vi "Begin - Davis.vi"(8 "error in":errorcluster) -> (0 "error out":errorcluster)   [LabVIEW 2018]
doc: "Called before other user functions, this VI is expected to open initial I/O refnums, load in file data, and do all program initialization. Notice that the <B>error out</B> terminal is simply used for data flow. Wiring it to other structures or subVIs ensures that this VI runs first."
uses:
  <vilib>/Rock Robotics/WPI/ThirdParty/Phoenix-LabVIEW/Motor Controller/Controls/CTRE_Phoenix_MotorControl_EnhancedMotorControllerConfigurables.ctl
  <vilib>/Rock Robotics/WPI/ThirdParty/Phoenix-LabVIEW/Motor Controller/Controls/CTRE_Phoenix_MotorControl_BaseConfigurables.ctl
  <vilib>/Rock Robotics/WPI/ThirdParty/Phoenix-LabVIEW/Motor Controller/Controls/CTRE_Phoenix_MotorControl_VelocityMeasurementPeriod.ctl
  <vilib>/Rock Robotics/WPI/ThirdParty/Phoenix-LabVIEW/Motor Controller/Controls/CTRE_Phoenix_MotorControl_SlotStructure.ctl
  <vilib>/Rock Robotics/WPI/ThirdParty/Phoenix-LabVIEW/Motor Controller/Controls/CTRE_Phoenix_MotorControl_FilterStruct.ctl
  <vilib>/Rock Robotics/WPI/ThirdParty/Phoenix-LabVIEW/Motor Controller/Controls/CTRE_Phoenix_MotorControl_RemoteSourceType.ctl
  <vilib>/Rock Robotics/WPI/ThirdParty/Phoenix-LabVIEW/Controls/CTRE_Phoenix_CustomParamConfiguration.ctl
  <vilib>/Rock Robotics/WPI/ThirdParty/Phoenix-LabVIEW/Motor Controller/Controls/CTRE_Phoenix_MotorControl_FeedbackDevice.ctl
  <vilib>/Rock Robotics/WPI/ThirdParty/Phoenix-LabVIEW/Motor Controller/Controls/CTRE_Phoenix_MotorControl_SensorTermFeedbackDevice_Enhanced.ctl
  <vilib>/Rock Robotics/WPI/ThirdParty/Phoenix-LabVIEW/Motor Controller/Controls/CTRE_Phoenix_MotorControl_LimitSwitchNormal.ctl
  <vilib>/Rock Robotics/WPI/ThirdParty/Phoenix-LabVIEW/Motor Controller/Controls/CTRE_Phoenix_MotorControl_LimitSwitchSource_Local.ctl
  <vilib>/Rock Robotics/WPI/DriverStation/WPI_DriverStationRobotMode2.ctl
  <vilib>/Rock Robotics/WPI/ThirdParty/Phoenix-LabVIEW/Motor Controller/Controls/CTRE_Phoenix_MotorControl_ControlMode.ctl
  <vilib>/Rock Robotics/WPI/Solenoid/WPI_SolenoidChannel.ctl
  <vilib>/Rock Robotics/WPI/SafetyOutput/WPI_SafetyOutputConfigMenu.ctl
  <vilib>/Rock Robotics/WPI/Joystick/WPI_JoystickDeviceEnum.ctl
  <vilib>/Rock Robotics/SystemInterfaces/DIO/FPGA_DIOPWMChannel.ctl
  <vilib>/Rock Robotics/SystemInterfaces/DIO/FPGA_DIOChannel.ctl
  Robot Global Data.vi
  <vilib>/Rock Robotics/Network Tables/NT Write String Array.vi
  <vilib>/Rock Robotics/WPI/Solenoid/WPI_SolenoidOpenDouble.vi
  <vilib>/Rock Robotics/WPI/Switch/WPI_SwitchOpenLimit.vi
  <vilib>/Rock Robotics/WPI/MotorControl/WPI_MotorControlOpen Victor.vi
  <vilib>/Rock Robotics/WPI/RobotDrive/WPI_RobotDriveOpen2MotorWithExistingMotors.vi
  <vilib>/Rock Robotics/WPI/MotorControl/WPI_MotorControlOpen SPARK.vi
  <vilib>/Rock Robotics/WPI/RobotDrive/WPI_RobotDriveOpen2MotorWithTalon.vi
panel:
  in  "Enhanced Motor Controller Configurables":T1={"Base Configurables"={"openLoopRamp"=0.0, "closedLoopRamp"=0.0, "peakOutputForward"=1.0, "peakOutputReverse"=-1.0, "nominalOutputForward"=0.0, "nominalOutputReverse"=0.0, "neutralDeadband"=0.04, "voltageCompSaturation"=0.0, "voltageMeasurementFilter"=32, "velocityMeasurementPeriod"=100, "velocityMeasurementWindow"=64, "forwardSoftLimitThreshold"=0, "reverseSoftLimitThreshold"=0, "forwardSoftLimitEnable"=FALSE, "reverseSoftLimitEnable"=FALSE, "slot0"={"P"=0.0, "I"=0.0, "D"=0.0, "F"=0.0, "integralZone"=0.0, "allowableClosedLoopError"=0, "maxIntegralAccumulator"=0.0, "closedLoopPeakOutput"=1.0, "closedLoopPeriod"=1}, "slot1"={"P"=0.0, "I"=0.0, "D"=0.0, "F"=0.0, "integralZone"=0.0, "allowableClosedLoopError"=0, "maxIntegralAccumulator"=0.0, "closedLoopPeakOutput"=1.0, "closedLoopPeriod"=1}, "slot2"={"P"=0.0, "I"=0.0, "D"=0.0, "F"=0.0, "integralZone"=0.0, "allowableClosedLoopError"=0, "maxIntegralAccumulator"=0.0, "closedLoopPeakOutput"=1.0, "closedLoopPeriod"=1}, "slot3"={"P"=0.0, "I"=0.0, "D"=0.0, "F"=0.0, "integralZone"=0.0, "allowableClosedLoopError"=0, "maxIntegralAccumulator"=0.0, "closedLoopPeakOutput"=1.0, "closedLoopPeriod"=1}, "auxPIDPolarity"=FALSE, "remoteFilter0"={"remoteSensorDeviceID"=0, "remoteSensorSource"=enum."Off"}, "remoteFilter1"={"remoteSensorDeviceID"=0, "remoteSensorSource"=enum."Off"}, "motionCruiseVelocity"=0, "motionAcceleration"=0, "motionProfileTrajectoryPeriod"=0, "feedbackNotContinuous"=FALSE, "remoteSensorClosedLoopDisableNeutralOnLOS"=FALSE, "clearPositionOnLimitF"=FALSE, "clearPositionOnLimitR"=FALSE, "clearPositionOnQuadIdx"=FALSE, "limitSwitchDisableNeutralOnLOS"=FALSE, "softLimitDisableNeutralOnLOS"=FALSE, "pulseWidthPeriod_EdgesPerRot"=1, "pulseWidthPeriod_FilterWindowSz"=1, "customParam"={"customParam0"=0, "customParam1"=0}, "trajectoryInterpolationEnable"=TRUE}, "primaryPID"={"selectedFeedbackCoefficient"=1.0, "selectedFeedbackSensor"=0}, "auxiliaryPID"={"selectedFeedbackCoefficient"=1.0, "selectedFeedbackSensor"=0}, "sum0Term"=0, "sum1Term"=0, "diff0Term"=0, "diff1Term"=0, "forwardLimitSwitchNormal"=enum."Normally Open", "reverseLimitSwitchNormal"=enum."Normally Open", "forwardLimitSwitchDeviceID"=0, "reverseLimitSwitchDeviceID"=0, "forwardLimitSwitchSource"=enum."Feedback Connector", "reverseLimitSwitchSource"=enum."Feedback Connector", "peakCurrentLimit"=1, "peakCurrentDuration"=1, "continuousCurrentLimit"=1} {"diff1Term" items=["QuadEncoder"=0, "Analog"=2, "Tachometer"=4, "Pulse Width Encoded Position"=8, "Remote Source 0"=11, "Remote Source 1"=12, "Software Emulated"=15]; "diff0Term" items=["QuadEncoder"=0, "Analog"=2, "Tachometer"=4, "Pulse Width Encoded Position"=8, "Remote Source 0"=11, "Remote Source 1"=12, "Software Emulated"=15]; "sum1Term" items=["QuadEncoder"=0, "Analog"=2, "Tachometer"=4, "Pulse Width Encoded Position"=8, "Remote Source 0"=11, "Remote Source 1"=12, "Software Emulated"=15]; "sum0Term" items=["QuadEncoder"=0, "Analog"=2, "Tachometer"=4, "Pulse Width Encoded Position"=8, "Remote Source 0"=11, "Remote Source 1"=12, "Software Emulated"=15]; "auxiliaryPID"."selectedFeedbackSensor" items=["QuadEncoder"=0, "Analog"=2, "Tachometer"=4, "Pulse Width Encoded Position"=8, "Sensor Sum (S0 + S1)"=9, "Sensor Difference (D0 - D1)"=10, "Remote Source 0"=11, "Remote Source 1"=12, "Software Emulated"=15]; "primaryPID"."selectedFeedbackSensor" items=["QuadEncoder"=0, "Analog"=2, "Tachometer"=4, "Pulse Width Encoded Position"=8, "Sensor Sum (S0 + S1)"=9, "Sensor Difference (D0 - D1)"=10, "Remote Source 0"=11, "Remote Source 1"=12, "Software Emulated"=15]; "Base Configurables"."velocityMeasurementPeriod" items=["Period_1ms"=1, "Period_2ms"=2, "Period_5ms"=5, "Period_10ms"=10, "Period_20ms"=20, "Period_25ms"=25, "Period_50ms"=50, "Period_100ms"=100]}
  # "Sum and Diff terms are ways to select more than one sensor as a feedback device. \n Sum 0 is the first feedback device to be used for the Sum term.\n Sum 1 is the feedback device to be added to Sum 0 for the Sum term.\n Diff 0 and Diff 1 work in a similar manner."
  # "These are only applicable\nif using a remote limit switch.\n\nLocal limit switches/no limit\nswitches do not use this."
  # "Current is below Continuous threshold AND\n\n(Requested output is weaker** than applied motor\noutput OR is in the opposite direction).\n/\nMotor output is set to requested output."
  # "Current is above Peak* Threshold for Peak Duration.\n/\nReduce motor output (towards neutral)."
  # "Current is below Continuous threshold.\n/\nRamp motor output towards requested output."
  # "Current is above Continuous threshold.\n/\nReduce motor output (towards neutral)."
  # "Current Limiting is NOT enabled\nby default.\nCall this VI to enable."
  # "*If the configured Peak Threshold is less than the Continuous Threshold, the applied Peak Threshold is set equal to the Configured Continuous Threshold in firmware.\n** Both requested output and applied motor output are in the same direction, and requested output is closer to neutral."
  # "False: Primary Output = PID[0] + PID[1]  ---  Auxiliary Output = PID[0] - PID[1]\nTrue:  Primary Output = PID[0] - PID[1] --- Auxiliary Output = PID[0] + PID[1]"
  # "Enable the motion profile executor to perform linear interpolation between profile points.  Defaults to True."
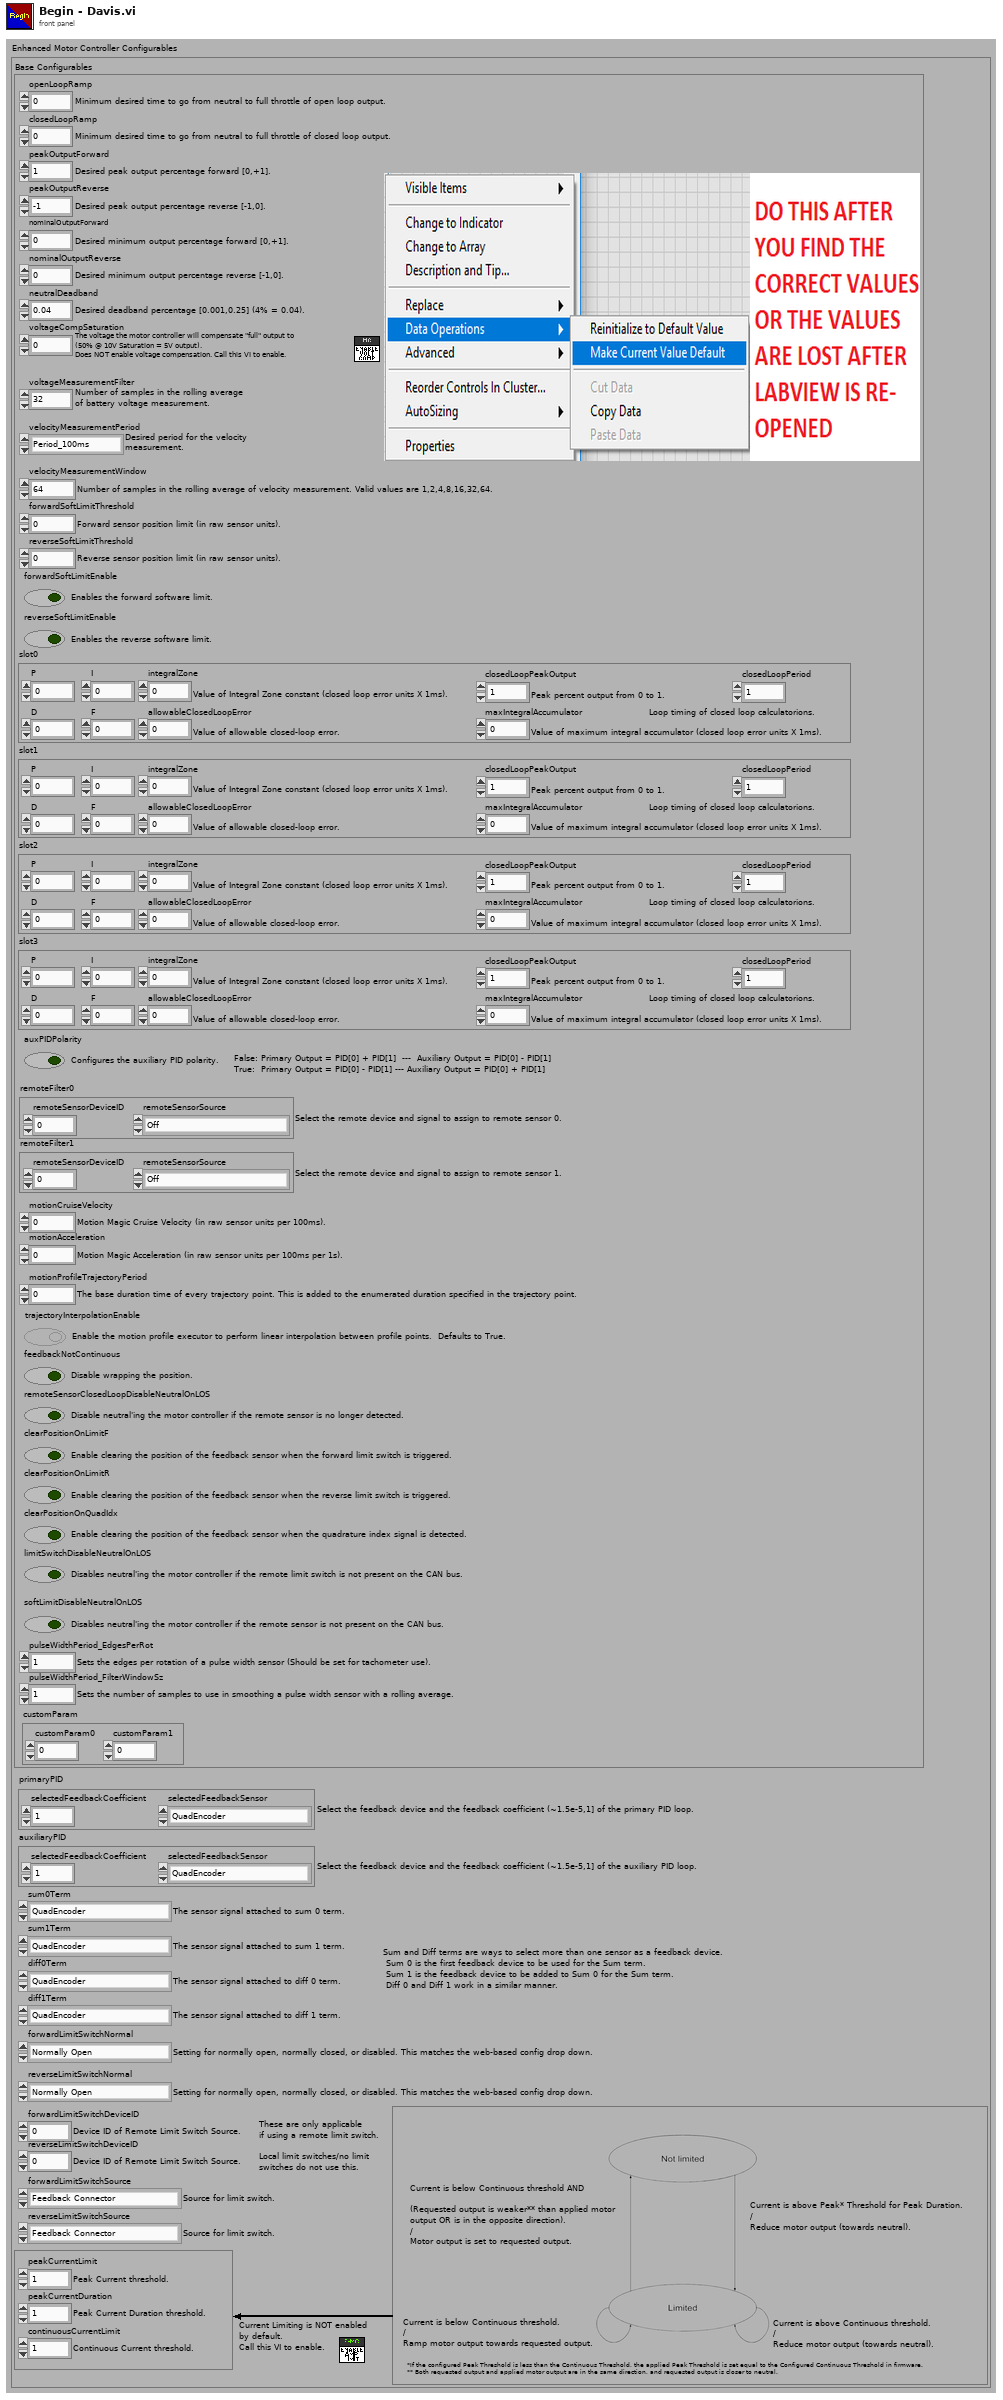
[diagram p1: front panel]
types:
  T1 = typedef "CTRE_Phoenix_MotorControl_EnhancedMotorControllerConfigurables.ctl" = cluster{"Base Configurables":T2, "primaryPID":cluster{"selectedFeedbackCoefficient":dbl, "selectedFeedbackSensor":T8}, "auxiliaryPID":cluster{"selectedFeedbackCoefficient":dbl, "selectedFeedbackSensor":T8}, "sum0Term":T9, "sum1Term":T9, "diff0Term":T9, "diff1Term":T9, "forwardLimitSwitchNormal":T10, "reverseLimitSwitchNormal":T10, "forwardLimitSwitchDeviceID":i32, "reverseLimitSwitchDeviceID":i32, "forwardLimitSwitchSource":T11, "reverseLimitSwitchSource":T11, "peakCurrentLimit":i32, "peakCurrentDuration":i32, "continuousCurrentLimit":i32}
  T2 = typedef "CTRE_Phoenix_MotorControl_BaseConfigurables.ctl" = cluster{"openLoopRamp":dbl, "closedLoopRamp":dbl, "peakOutputForward":dbl, "peakOutputReverse":dbl, "nominalOutputForward":dbl, "nominalOutputReverse":dbl, "neutralDeadband":dbl, "voltageCompSaturation":dbl, "voltageMeasurementFilter":i32, "velocityMeasurementPeriod":T3, "velocityMeasurementWindow":i32, "forwardSoftLimitThreshold":i32, "reverseSoftLimitThreshold":i32, "forwardSoftLimitEnable":bool, "reverseSoftLimitEnable":bool, "slot0":T4, "slot1":T4, "slot2":T4, "slot3":T4, "auxPIDPolarity":bool, "remoteFilter0":T5, "remoteFilter1":T5, "motionCruiseVelocity":i32, "motionAcceleration":i32, "motionProfileTrajectoryPeriod":i32, "feedbackNotContinuous":bool, "remoteSensorClosedLoopDisableNeutralOnLOS":bool, "clearPositionOnLimitF":bool, "clearPositionOnLimitR":bool, "clearPositionOnQuadIdx":bool, "limitSwitchDisableNeutralOnLOS":bool, "softLimitDisableNeutralOnLOS":bool, "pulseWidthPeriod_EdgesPerRot":i32, "pulseWidthPeriod_FilterWindowSz":i32, "customParam":T7, "trajectoryInterpolationEnable":bool}
  T3 = typedef "CTRE_Phoenix_MotorControl_VelocityMeasurementPeriod.ctl" = u16
  T4 = typedef "CTRE_Phoenix_MotorControl_SlotStructure.ctl" = cluster{"P":dbl, "I":dbl, "D":dbl, "F":dbl, "integralZone":dbl, "allowableClosedLoopError":i32, "maxIntegralAccumulator":dbl, "closedLoopPeakOutput":dbl, "closedLoopPeriod":i32}
  T5 = typedef "CTRE_Phoenix_MotorControl_FilterStruct.ctl" = cluster{"remoteSensorDeviceID":u8, "remoteSensorSource":T6}
  T6 = typedef "CTRE_Phoenix_MotorControl_RemoteSourceType.ctl" = enum16{"Off", "Talon SRX Selected Sensor", "Pigeon IMU Yaw", "Pigeon IMU Pitch", "Pigeon IMU Roll", "CANifier Quadrature", "CANifier PWM Input 0", "CANifier PWM Input 1", "CANifier PWM Input 2", "CANifier PWM Input 3", "Gadgeteer Pigeon Yaw", "Gadgeteer Pigeon Pitch", "Gadgeteer Pigeon Roll"}
  T7 = typedef "CTRE_Phoenix_CustomParamConfiguration.ctl" = cluster{"customParam0":i32, "customParam1":i32}
  T8 = typedef "CTRE_Phoenix_MotorControl_FeedbackDevice.ctl" = i8
  T9 = typedef "CTRE_Phoenix_MotorControl_SensorTermFeedbackDevice_Enhanced.ctl" = i8
  T10 = typedef "CTRE_Phoenix_MotorControl_LimitSwitchNormal.ctl" = enum16{"Normally Open", "Normally Closed", "Disabled"}
  T11 = typedef "CTRE_Phoenix_MotorControl_LimitSwitchSource_Local.ctl" = enum16{"Feedback Connector", "Remote Talon SRX", "Remote CANifier", "Deactivated"}
  T12 = typedef "WPI_SafetyOutputConfigMenu.ctl" = enum16{"Enable", "Disable"}
  T13 = typedef "WPI_SolenoidChannel.ctl" = enum8{"Solenoid 0", "Solenoid 1", "Solenoid 2", "Solenoid 3", "Solenoid 4", "Solenoid 5", "Solenoid 6", "Solenoid 7", "Invalid"}
  T14 = typedef "FPGA_DIOPWMChannel.ctl" = enum8{"PWM 0", "PWM 1", "PWM 2", "PWM 3", "PWM 4", "PWM 5", "PWM 6", "PWM 7", "PWM 8", "PWM 9", "PWM MXP 0", "PWM MXP 1", "PWM MXP 2", "PWM MXP 3", "PWM MXP 4", "PWM MXP 5", "PWM MXP 6", "PWM MXP 7", "PWM MXP 8", "PWM MXP 9", "Invalid"}
  T15 = typedef "WPI_JoystickDeviceEnum.ctl" = enum16{"USB 0", "USB 1", "USB 2", "USB 3", "USB 4", "USB 5"}
  T16 = typedef "FPGA_DIOChannel.ctl" = enum8{"DIO 0", "DIO 1", "DIO 2", "DIO 3", "DIO 4", "DIO 5", "DIO 6", "DIO 7", "DIO 8", "DIO 9", "DIO MXP 0", "DIO MXP 1", "DIO MXP 2", "DIO MXP 3", "DIO MXP 4", "DIO MXP 5", "DIO MXP 6", "DIO MXP 7", "DIO MXP 8", "DIO MXP 9", "DIO MXP 10", "DIO MXP 11", "DIO MXP 12", "DIO MXP 13", "DIO MXP 14", "DIO MXP 15", "SPI Port CS1", "SPI Port CS2", "SPI Port CS3", "SPI Port MISO", "SPI Port MOSI", "Invalid"}
  T17 = typedef "CTRE_Phoenix_MotorControl_ControlMode.ctl" = u16
  T18 = typedef "WPI_DriverStationRobotMode2.ctl" = enum16{"Autonomous Disabled", "Autonomous Enabled", "Teleop Disabled", "Teleop Enabled", "Disconnected", "Finish", "Test Disabled", "Test Enabled", "Emergency Stopped"}
  T19 = typedef "WPI_JoystickDevRef.ctl" = cluster{"Device":T15}
  T20 = typedef "WPI_RobotDriveDevRef.ctl" = cluster{"DevStatus":errorcluster, "Motors[]":T21[], "Square Inputs":bool, "Max Output":dbl}
  T21 = typedef "WPI_MotorControlDeviceRef.ctl" = cluster{"DeviceStatus":errorcluster, "Type":T22, "PWM":cluster{"PWM Channel":T14, "DeadBand":T23}, "CAN":cluster{"Device Number":u8, "SetOutput VI Ref":variant, "GetOutput VI Ref":variant, "Enable VI Ref":variant, "Disable VI Ref":variant, "Data":variant}, "Invert":bool, "DIO PWM":cluster{"PWM \"Enable\" Channel":T14, "DIOChannel":T16, "PWM Rate":dbl}}
  T22 = typedef "WPI_MotorControlType.ctl" = enum16{"PWM", "CAN", "DIO PWM"}
  T23 = typedef "WPI_PWMDeadband.ctl" = cluster{"Name":string, "maxPositivePwm":i32, "minPositivePwm":i32, "centerPwm":i32, "maxNegativePwm":i32, "minNegativePwm":i32, "angularRange":u16}
  T24 = typedef "WPI_SwitchDevRef.ctl" = cluster{"DevStatus":errorcluster, "DIO Channel":T16, "CntIndex":T25, "Normally Closed":bool}
  T25 = typedef "FPGA_CounterCtrSystemIndex.ctl" = enum8{"Ctr 0", "Ctr 1", "Ctr 2", "Ctr 3", "Ctr 4", "Ctr 5", "Ctr 6", "Ctr 7", "Invalid"}
  T26 = typedef "WPI_ServoDeviceRef.ctl" = cluster{"DeviceStatus":errorcluster, "PWM Channel":T14, "DeadBand":T23}
  T27 = typedef "WPI_SolenoidDevRef.ctl" = cluster{"DevStatus":errorcluster, "Pneumatics Control Module":u8, "Forward Solenoid Channel":T13, "Reverse Solenoid Channel":T13}
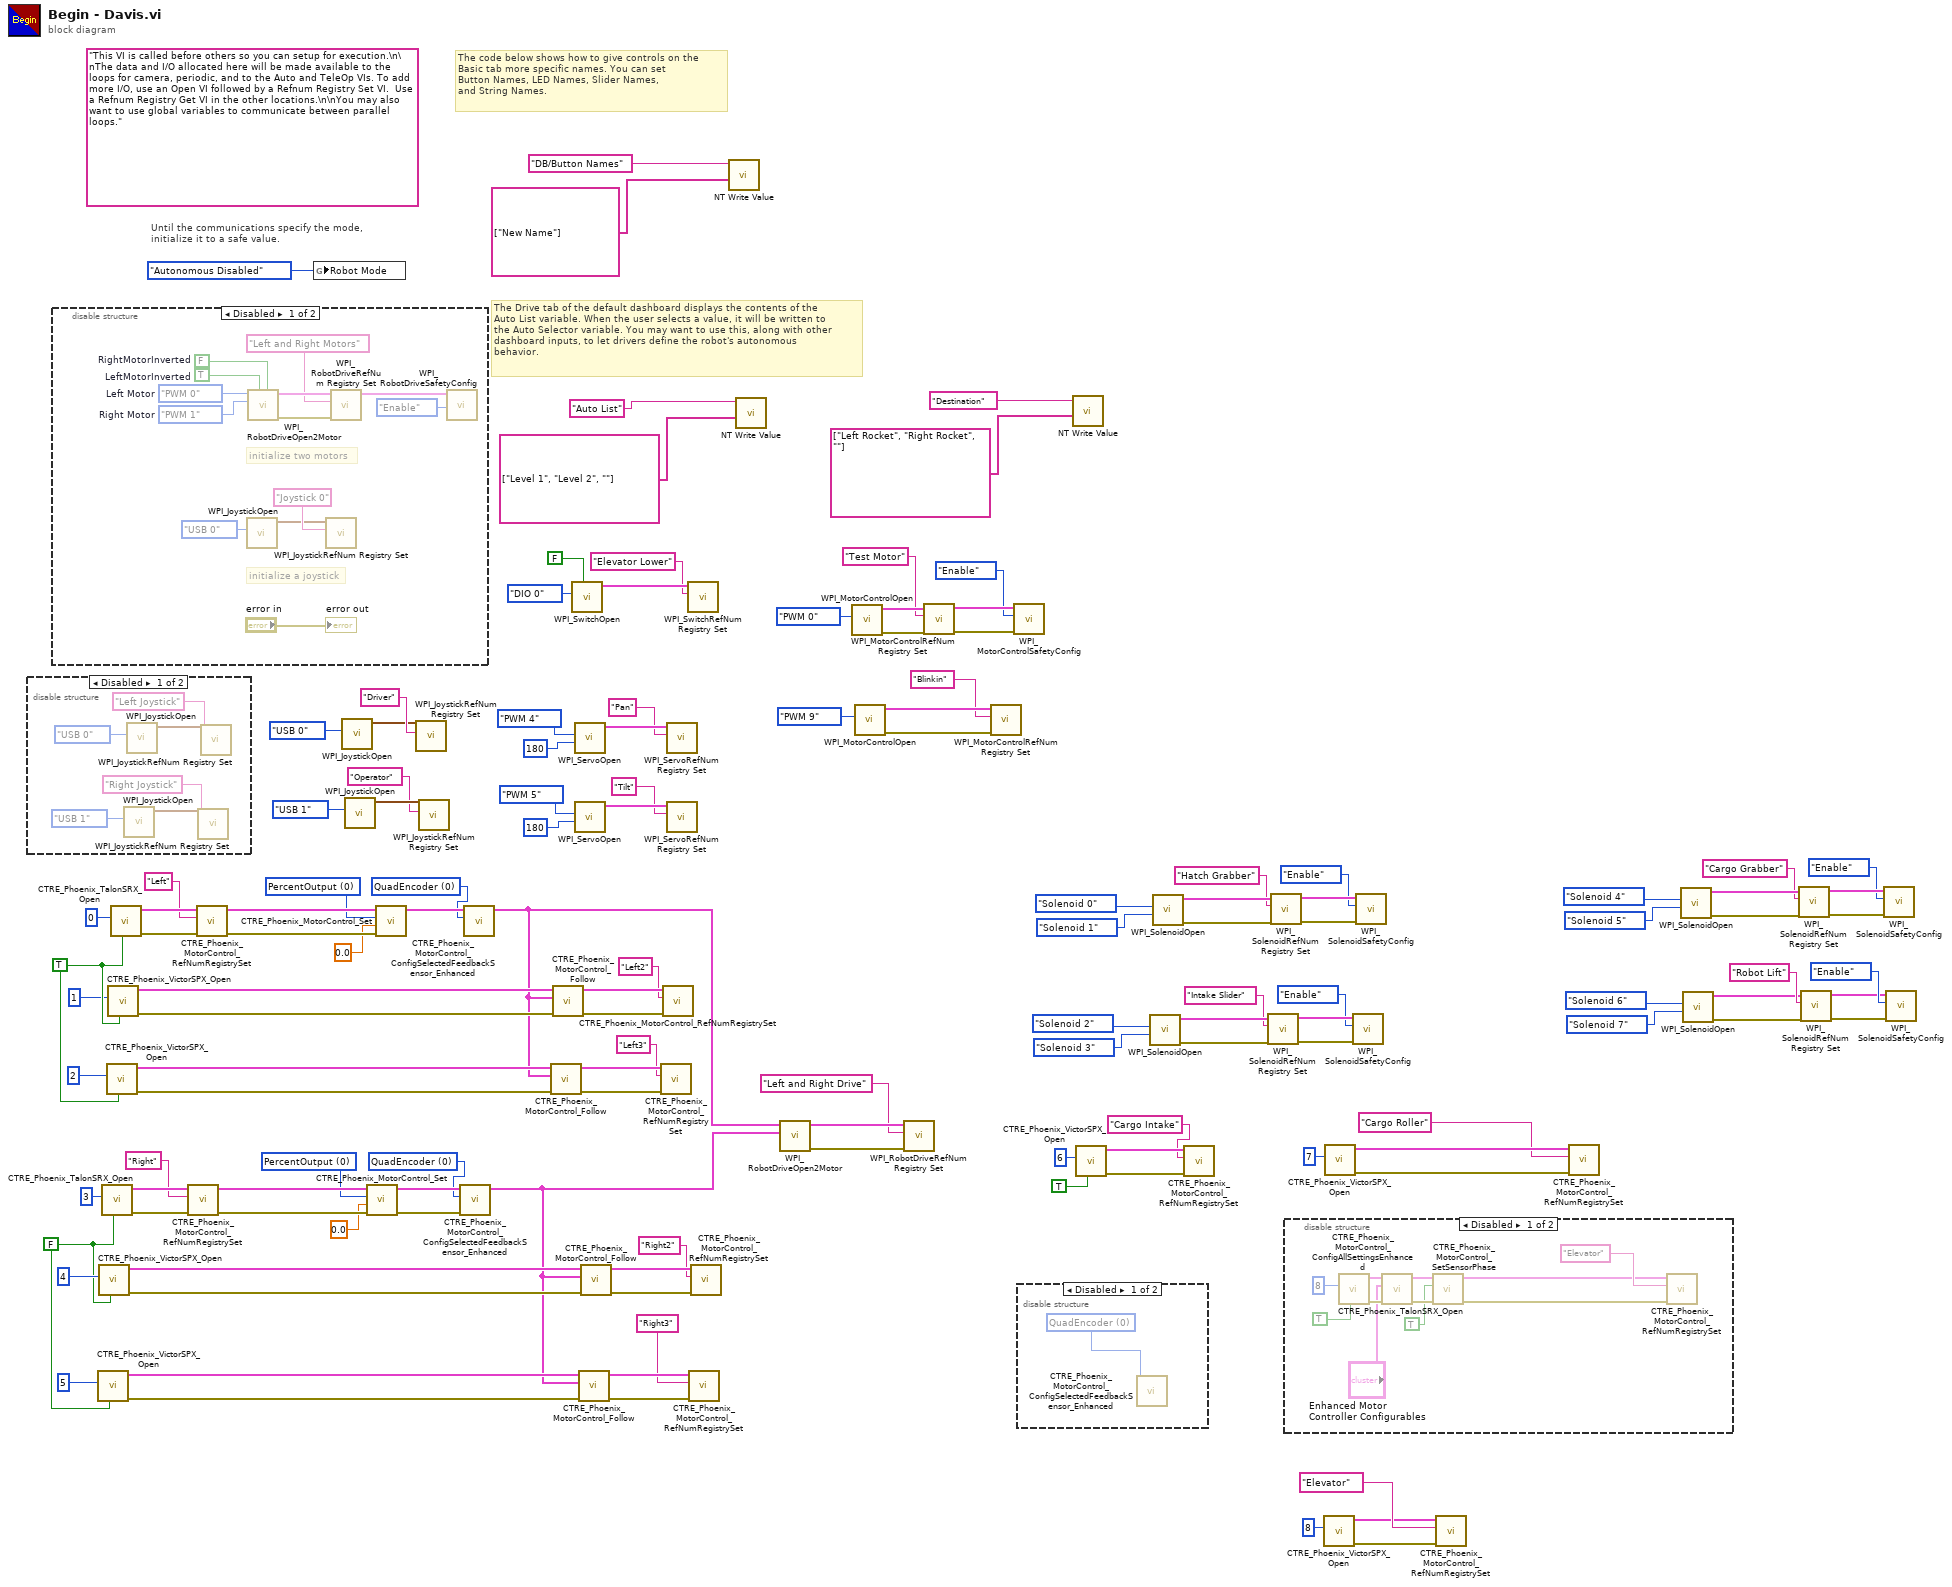
[diagram p0: block diagram]
diagram:
  w20 = T8 0 items=["QuadEncoder"=0, "Analog"=2, "Tachometer"=4, "Pulse Width Encoded Position"=8, "Sensor Sum (S0 + S1)"=9, "Sensor Difference (D0 - D1)"=10, "Remote Source 0"=11, "Remote Source 1"=12, "Software Emulated"=15] ("Feedback Device")
  w23 = T8 0 items=["QuadEncoder"=0, "Analog"=2, "Tachometer"=4, "Pulse Width Encoded Position"=8, "Sensor Sum (S0 + S1)"=9, "Sensor Difference (D0 - D1)"=10, "Remote Source 0"=11, "Remote Source 1"=12, "Software Emulated"=15] ("Feedback Device")
  w90 = T17 0 items=["PercentOutput"=0, "Position"=1, "Velocity"=2, "Current"=3, "Follower"=5, "MotionProfile"=6, "MotionMagic"=7, "MotionProfileArc"=10, "Disabled"=15] ("Control Mode")
  w91 = T17 0 items=["PercentOutput"=0, "Position"=1, "Velocity"=2, "Current"=3, "Follower"=5, "MotionProfile"=6, "MotionMagic"=7, "MotionProfileArc"=10, "Disabled"=15] ("Control Mode")
  w43 = FALSE ("Invert")
  w126 = TRUE ("Invert")
  (unwired) "This VI is called before others so you can setup for execution.\n\nThe data and I/O allocated here will be made available to the loops for camera, periodic, and to the Auto and TeleOp VIs. To add more I/O, use an Open VI followed by a Refnum Registry Set VI.  Use a Refnum Registry Get VI in the other locations.\n\nYou may also want to use global variables to communicate between parallel loops."
  # "The Drive tab of the default dashboard displays the contents of the\nAuto List variable. When the user selects a value, it will be written to\nthe Auto Selector variable. You may want to use this, along with other\ndashboard inputs, to let drivers define the robot's autonomous\nbehavior."
  # "The code below shows how to give controls on the\nBasic tab more specific names. You can set\nButton Names, LED Names, Slider Names,\nand String Names."
  # "Until the communications specify the mode,\ninitialize it to a safe value."
  n1 = disable-structure shown="Disabled" {
    frame Disabled {
      n2 = call <vilib>:"WPI_JoystickOpen.vi"("JoystickDevice"=WPI_JoystickDeviceEnum."USB 1") -> ("JoystickDevRef"=w136:T19)  [unwired: 10 in]
      n3 = call <vilib>:"WPI_JoystickOpen.vi"("JoystickDevice"=WPI_JoystickDeviceEnum."USB 0") -> ("JoystickDevRef"=w139:T19)  [unwired: 10 in]
      n4 = call <vilib>:"WPI_JoystickRefNum Registry Set.vi"("refnum name"="Right Joystick", "JoystickDevRef"=w136) -> ()  [unwired: 8 in, 2 out]
      n5 = call <vilib>:"WPI_JoystickRefNum Registry Set.vi"("refnum name"="Left Joystick", "JoystickDevRef"=w139) -> ()  [unwired: 8 in, 2 out]
    }
    frame Enabled {
    }
  }
  n6 = disable-structure shown="Disabled" {
    frame Disabled {
      w146 = FPGA_DIOPWMChannel."PWM 1"  # Right Motor
      w147 = FPGA_DIOPWMChannel."PWM 0"  # Left Motor
      w151 = TRUE  # LeftMotorInverted
      w152 = FALSE  # RightMotorInverted
      # "initialize a joystick"
      # "initialize two motors"
      n7 = call <vilib>:"WPI_JoystickOpen.vi"("JoystickDevice"=WPI_JoystickDeviceEnum."USB 0") -> ("JoystickDevRef"=w142:T19)  [unwired: 10 in]
      n8 = call-poly <vilib>:"WPI_RobotDriveOpen2Motor.vi"("Right Motor Inverted"=w152, "Left Motor Inverted"=w151, "Right Motor"=w146, "Left Motor"=w147) -> ("error out"=w148:errorcluster, "RobotDriveDevRef"=w150:T20)  [unwired: 1 in, 5 out]
      n9 = call <vilib>:"WPI_JoystickRefNum Registry Set.vi"("refnum name"="Joystick 0", "JoystickDevRef"=w142) -> ()  [unwired: 8 in, 2 out]
      n10 = call <vilib>:"WPI_RobotDriveRefNum Registry Set.vi"("error in (no error)"=w148, "refnum name"="Left and Right Motors", "RobotDriveDevRef"=w150) -> ("RobotDriveDevRef"=w145:T20)  [unwired: 1 in, 7 out]
      n11 = call <vilib>:"WPI_RobotDriveSafetyConfig.vi"("mode"=WPI_SafetyOutputConfigMenu."Enable", "RobotDriveDevRef"=w145) -> ()  [unwired: 8 in, 2 out]
      "error out" <- "error in"
    }
    frame Enabled {
    }
  }
  n12 = call <vilib>:"CTRE_Phoenix_VictorSPX_Open.vi"("Invert"=w43, "Device Number"=u8 5) -> ("error out"=w99:errorcluster, "CAN Talon SRX Ref"=w104:T21)  [unwired: 8 in]
  n13 = call <vilib>:"CTRE_Phoenix_VictorSPX_Open.vi"("Invert"=w43, "Device Number"=u8 4) -> ("error out"=w101:errorcluster, "CAN Talon SRX Ref"=w109:T21)  [unwired: 8 in]
  n14 = call <vilib>:"CTRE_Phoenix_TalonSRX_Open.vi"("Invert"=w43, "Device Number"=u8 3) -> ("error out"=w103:errorcluster, "CAN Talon SRX Ref"=w112:T21)  [unwired: 8 in]
  n15 = call <vilib>:"CTRE_Phoenix_VictorSPX_Open.vi"("Invert"=w126, "Device Number"=u8 2) -> ("error out"=w114:errorcluster, "CAN Talon SRX Ref"=w119:T21)  [unwired: 8 in]
  n16 = call <vilib>:"CTRE_Phoenix_VictorSPX_Open.vi"("Invert"=w126, "Device Number"=u8 1) -> ("error out"=w116:errorcluster, "CAN Talon SRX Ref"=w124:T21)  [unwired: 8 in]
  n17 = call <vilib>:"CTRE_Phoenix_TalonSRX_Open.vi"("Invert"=w126, "Device Number"=u8 0) -> ("error out"=w118:errorcluster, "CAN Talon SRX Ref"=w128:T21)  [unwired: 8 in]
  n18 = call <vilib>:"CTRE_Phoenix_MotorControl_RefNumRegistrySet.vi"("error in (no error)"=w103, "refnum name"="Right", "PhoenixMotorControlDevRef"=w112) -> ("error out"=w102:errorcluster, "PhoenixMotorControlDevRef"=w110:T21)  [unwired: 7 in]
  n19 = call <vilib>:"CTRE_Phoenix_MotorControl_RefNumRegistrySet.vi"("error in (no error)"=w118, "refnum name"="Left", "PhoenixMotorControlDevRef"=w128) -> ("error out"=w117:errorcluster, "PhoenixMotorControlDevRef"=w125:T21)  [unwired: 7 in]
  n20 = global write "Robot Global Data.vi" "Robot Mode"(WPI_DriverStationRobotMode2."Autonomous Disabled" ("Robot Mode")) -> ()
  n21 = call <vilib>:"WPI_JoystickOpen.vi"("JoystickDevice"=WPI_JoystickDeviceEnum."USB 0") -> ("JoystickDevRef"=w30:T19)  [unwired: 10 in]
  n22 = call <vilib>:"WPI_JoystickOpen.vi"("JoystickDevice"=WPI_JoystickDeviceEnum."USB 1") -> ("JoystickDevRef"=w63:T19)  [unwired: 10 in]
  n23 = call <vilib>:"CTRE_Phoenix_MotorControl_Set.vi"("error in (no error)"=w102, "Output"=0.0, "Control Mode"=w90, "PhoenixMotorControlDevRef"=w110) -> ("error out"=w24:errorcluster, "PhoenixMotorControlDevRef"=w26:T21)  [unwired: 6 in]
  n24 = call <vilib>:"CTRE_Phoenix_MotorControl_Set.vi"("error in (no error)"=w117, "Output"=0.0, "Control Mode"=w91, "PhoenixMotorControlDevRef"=w125) -> ("PhoenixMotorControlDevRef"=w22:T21)  [unwired: 6 in, 1 out]
  n25 = call <vilib>:"WPI_JoystickRefNum Registry Set.vi"("refnum name"="Driver", "JoystickDevRef"=w30) -> ()  [unwired: 8 in, 2 out]
  n26 = call <vilib>:"WPI_JoystickRefNum Registry Set.vi"("refnum name"="Operator", "JoystickDevRef"=w63) -> ()  [unwired: 8 in, 2 out]
  n27 = call <vilib>:"CTRE_Phoenix_MotorControl_ConfigSelectedFeedbackSensor_Enhanced.vi"("error in (no error)"=w24, "Feedback Device"=w23, "PhoenixMotorControlDevRef"=w26) -> ("PhoenixMotorControlDevRef"=w25:T21)  [unwired: 7 in, 1 out]
  n28 = call <vilib>:"CTRE_Phoenix_MotorControl_ConfigSelectedFeedbackSensor_Enhanced.vi"("Feedback Device"=w20, "PhoenixMotorControlDevRef"=w22) -> ("PhoenixMotorControlDevRef"=w21:T21)  [unwired: 8 in, 1 out]
  n29 = call <vilib>:"CTRE_Phoenix_MotorControl_Follow.vi"("error in (no error)"=w114, "Master Controller to Follow"=w21, "PhoenixMotorControlDevRef"=w119) -> ("error out"=w113:errorcluster, "PhoenixMotorControlDevRef"=w121:T21)  [unwired: 7 in]
  n30 = call <vilib>:"CTRE_Phoenix_MotorControl_Follow.vi"("error in (no error)"=w116, "Master Controller to Follow"=w21, "PhoenixMotorControlDevRef"=w124) -> ("error out"=w115:errorcluster, "PhoenixMotorControlDevRef"=w123:T21)  [unwired: 7 in]
  n31 = call-poly <vilib>:"WPI_SwitchOpen.vi"("Normally Closed"=FALSE, "DIO Channel"=FPGA_DIOChannel."DIO 0") -> ("SwitchDevRef"=w52:T24)  [unwired: 8 in, 1 out]
  n32 = call <vilib>:"WPI_ServoOpen.vi"("Angular Range"=u16 180, "PWM Channel"=FPGA_DIOPWMChannel."PWM 4") -> ("ServoDeviceRef"=w59:T26)  [unwired: 8 in, 1 out]
  n33 = call <vilib>:"WPI_ServoOpen.vi"("Angular Range"=u16 180, "PWM Channel"=FPGA_DIOPWMChannel."PWM 5") -> ("ServoDeviceRef"=w56:T26)  [unwired: 8 in, 1 out]
  n34 = call <vilib>:"CTRE_Phoenix_MotorControl_Follow.vi"("error in (no error)"=w99, "Master Controller to Follow"=w25, "PhoenixMotorControlDevRef"=w104) -> ("error out"=w98:errorcluster, "PhoenixMotorControlDevRef"=w106:T21)  [unwired: 7 in]
  n35 = call <vilib>:"CTRE_Phoenix_MotorControl_Follow.vi"("error in (no error)"=w101, "Master Controller to Follow"=w25, "PhoenixMotorControlDevRef"=w109) -> ("error out"=w100:errorcluster, "PhoenixMotorControlDevRef"=w108:T21)  [unwired: 7 in]
  n36 = call <vilib>:"CTRE_Phoenix_MotorControl_RefNumRegistrySet.vi"("error in (no error)"=w113, "refnum name"="Left3", "PhoenixMotorControlDevRef"=w121) -> ()  [unwired: 7 in, 2 out]
  n37 = call <vilib>:"CTRE_Phoenix_MotorControl_RefNumRegistrySet.vi"("error in (no error)"=w115, "refnum name"="Left2", "PhoenixMotorControlDevRef"=w123) -> ()  [unwired: 7 in, 2 out]
  n38 = call <vilib>:"WPI_ServoRefNum Registry Set.vi"("refnum name"="Pan", "ServoDeviceRef"=w59) -> ()  [unwired: 8 in, 2 out]
  n39 = call <vilib>:"WPI_ServoRefNum Registry Set.vi"("refnum name"="Tilt", "ServoDeviceRef"=w56) -> ()  [unwired: 8 in, 2 out]
  n40 = call <vilib>:"WPI_SwitchRefNum Registry Set.vi"("refnum name"="Elevator Lower", "SwitchDevRef"=w52) -> ()  [unwired: 8 in, 2 out]
  n41 = call <vilib>:"CTRE_Phoenix_MotorControl_RefNumRegistrySet.vi"("error in (no error)"=w98, "refnum name"="Right3", "PhoenixMotorControlDevRef"=w106) -> ()  [unwired: 7 in, 2 out]
  n42 = call <vilib>:"CTRE_Phoenix_MotorControl_RefNumRegistrySet.vi"("error in (no error)"=w100, "refnum name"="Right2", "PhoenixMotorControlDevRef"=w108) -> ()  [unwired: 7 in, 2 out]
  n43 = call-poly <vilib>:"NT Write Value.vi"("String Array"=string[] ["New Name"], "Name"="DB/Button Names") -> ()  [unwired: 9 in, 1 out]
  n44 = call-poly <vilib>:"NT Write Value.vi"("String Array"=string[] ["Level 1", "Level 2", ""], "Name"="Auto List") -> ()  [unwired: 9 in, 1 out]
  n45 = call-poly <vilib>:"WPI_RobotDriveOpen2Motor.vi"("Right Motor Dev Ref"=w25, "Left Motor Dev Ref"=w21) -> ("error out"=w27:errorcluster, "RobotDriveDevRef"=w29:T20)  [unwired: 8 in]
  n46 = call-poly <vilib>:"WPI_MotorControlOpen.vi"("PWM Channel"=FPGA_DIOPWMChannel."PWM 0") -> ("error out"=w46:errorcluster, "MotorControlDeviceRef"=w49:T21)  [unwired: 9 in]
  n47 = call-poly <vilib>:"WPI_MotorControlOpen.vi"("PWM Channel"=FPGA_DIOPWMChannel."PWM 9") -> ("error out"=w14:errorcluster, "MotorControlDeviceRef"=w15:T21)  [unwired: 9 in]
  n48 = call <vilib>:"WPI_RobotDriveRefNum Registry Set.vi"("error in (no error)"=w27, "refnum name"="Left and Right Drive", "RobotDriveDevRef"=w29) -> ()  [unwired: 7 in, 2 out]
  n49 = call <vilib>:"WPI_MotorControlRefNum Registry Set.vi"("error in (no error)"=w46, "refnum name"="Test Motor", "MotorControlDevRef"=w49) -> ("error out"=w45:errorcluster, "MotorControlDevRef"=w47:T21)  [unwired: 7 in]
  n50 = call <vilib>:"WPI_MotorControlRefNum Registry Set.vi"("error in (no error)"=w14, "refnum name"="Blinkin", "MotorControlDevRef"=w15) -> ()  [unwired: 7 in, 2 out]
  n51 = call <vilib>:"WPI_MotorControlSafetyConfig.vi"("error in (no error)"=w45, "mode"=WPI_SafetyOutputConfigMenu."Enable", "MotorControlDevRef"=w47) -> ()  [unwired: 7 in, 2 out]
  n52 = disable-structure shown="Disabled" {
    frame Disabled {
      w153 = T8 0 items=["QuadEncoder"=0, "Analog"=2, "Tachometer"=4, "Pulse Width Encoded Position"=8, "Sensor Sum (S0 + S1)"=9, "Sensor Difference (D0 - D1)"=10, "Remote Source 0"=11, "Remote Source 1"=12, "Software Emulated"=15] ("Feedback Device")
      n53 = call <vilib>:"CTRE_Phoenix_MotorControl_ConfigSelectedFeedbackSensor_Enhanced.vi"("Feedback Device"=w153) -> ()  [unwired: 9 in, 2 out]
    }
    frame Enabled {
    }
  }
  n54 = call-poly <vilib>:"NT Write Value.vi"("String Array"=string[] ["Left Rocket", "Right Rocket", ""], "Name"="Destination") -> ()  [unwired: 9 in, 1 out]
  n55 = call <vilib>:"CTRE_Phoenix_VictorSPX_Open.vi"("Invert"=TRUE, "Device Number"=u8 6) -> ("error out"=w40:errorcluster, "CAN Talon SRX Ref"=w41:T21)  [unwired: 8 in]
  n56 = call-poly <vilib>:"WPI_SolenoidOpen.vi"("Reverse Solenoid Channel"=WPI_SolenoidChannel."Solenoid 3", "Forward Solenoid Channel"=WPI_SolenoidChannel."Solenoid 2") -> ("error out"=w75:errorcluster, "SolenoidDevRef"=w77:T27)  [unwired: 8 in]
  n57 = call-poly <vilib>:"WPI_SolenoidOpen.vi"("Reverse Solenoid Channel"=WPI_SolenoidChannel."Solenoid 1", "Forward Solenoid Channel"=WPI_SolenoidChannel."Solenoid 0") -> ("error out"=w83:errorcluster, "SolenoidDevRef"=w85:T27)  [unwired: 8 in]
  n58 = call <vilib>:"CTRE_Phoenix_MotorControl_RefNumRegistrySet.vi"("error in (no error)"=w40, "refnum name"="Cargo Intake", "PhoenixMotorControlDevRef"=w41) -> ()  [unwired: 7 in, 2 out]
  n59 = call <vilib>:"WPI_SolenoidRefNum Registry Set.vi"("error in (no error)"=w75, "refnum name"="Intake Slider", "SolenoidDevRef"=w77) -> ("error out"=w73:errorcluster, "SolenoidDevRef"=w74:T27)  [unwired: 7 in]
  n60 = call <vilib>:"WPI_SolenoidRefNum Registry Set.vi"("error in (no error)"=w83, "refnum name"="Hatch Grabber", "SolenoidDevRef"=w85) -> ("error out"=w81:errorcluster, "SolenoidDevRef"=w82:T27)  [unwired: 7 in]
  n61 = disable-structure shown="Disabled" {
    frame Disabled {
      n62 = call <vilib>:"CTRE_Phoenix_TalonSRX_Open.vi"("Invert"=TRUE, "Device Number"=u8 8) -> ("error out"=w160:errorcluster, "CAN Talon SRX Ref"=w161:T21)  [unwired: 8 in]
      n63 = call <vilib>:"CTRE_Phoenix_MotorControl_ConfigAllSettingsEnhanced.vi"("error in (no error)"=w160, "Enhanced Motor Controller Configurables"="Enhanced Motor Controller Configurables", "PhoenixMotorControlDevRef"=w161) -> ("error out"=w158:errorcluster, "PhoenixMotorControlDevRef"=w159:T21)  [unwired: 7 in]
      n64 = call <vilib>:"CTRE_Phoenix_MotorControl_SetSensorPhase.vi"("error in (no error)"=w158, "PhaseSensor"=TRUE, "PhoenixMotorControlDevRef"=w159) -> ("error out"=w156:errorcluster, "PhoenixMotorControlDevRef"=w157:T21)  [unwired: 7 in]
      n65 = call <vilib>:"CTRE_Phoenix_MotorControl_RefNumRegistrySet.vi"("error in (no error)"=w156, "refnum name"="Elevator", "PhoenixMotorControlDevRef"=w157) -> ()  [unwired: 7 in, 2 out]
    }
    frame Enabled {
    }
  }
  n66 = call <vilib>:"CTRE_Phoenix_VictorSPX_Open.vi"("Device Number"=u8 8) -> ("error out"=w3:errorcluster, "CAN Talon SRX Ref"=w2:T21)  [unwired: 9 in]
  n67 = call <vilib>:"CTRE_Phoenix_VictorSPX_Open.vi"("Device Number"=u8 7) -> ("error out"=w36:errorcluster, "CAN Talon SRX Ref"=w37:T21)  [unwired: 9 in]
  n68 = call <vilib>:"WPI_SolenoidSafetyConfig.vi"("error in (no error)"=w73, "mode"=WPI_SafetyOutputConfigMenu."Enable", "SolenoidDevRef"=w74) -> ()  [unwired: 7 in, 2 out]
  n69 = call <vilib>:"WPI_SolenoidSafetyConfig.vi"("error in (no error)"=w81, "mode"=WPI_SafetyOutputConfigMenu."Enable", "SolenoidDevRef"=w82) -> ()  [unwired: 7 in, 2 out]
  n70 = call <vilib>:"CTRE_Phoenix_MotorControl_RefNumRegistrySet.vi"("error in (no error)"=w3, "refnum name"="Elevator", "PhoenixMotorControlDevRef"=w2) -> ()  [unwired: 7 in, 2 out]
  n71 = call <vilib>:"CTRE_Phoenix_MotorControl_RefNumRegistrySet.vi"("error in (no error)"=w36, "refnum name"="Cargo Roller", "PhoenixMotorControlDevRef"=w37) -> ()  [unwired: 7 in, 2 out]
  n72 = call-poly <vilib>:"WPI_SolenoidOpen.vi"("Reverse Solenoid Channel"=WPI_SolenoidChannel."Solenoid 5", "Forward Solenoid Channel"=WPI_SolenoidChannel."Solenoid 4") -> ("error out"=w67:errorcluster, "SolenoidDevRef"=w69:T27)  [unwired: 8 in]
  n73 = call-poly <vilib>:"WPI_SolenoidOpen.vi"("Reverse Solenoid Channel"=WPI_SolenoidChannel."Solenoid 7", "Forward Solenoid Channel"=WPI_SolenoidChannel."Solenoid 6") -> ("error out"=w9:errorcluster, "SolenoidDevRef"=w7:T27)  [unwired: 8 in]
  n74 = call <vilib>:"WPI_SolenoidRefNum Registry Set.vi"("error in (no error)"=w67, "refnum name"="Cargo Grabber", "SolenoidDevRef"=w69) -> ("error out"=w65:errorcluster, "SolenoidDevRef"=w66:T27)  [unwired: 7 in]
  n75 = call <vilib>:"WPI_SolenoidRefNum Registry Set.vi"("error in (no error)"=w9, "refnum name"="Robot Lift", "SolenoidDevRef"=w7) -> ("error out"=w11:errorcluster, "SolenoidDevRef"=w10:T27)  [unwired: 7 in]
  n76 = call <vilib>:"WPI_SolenoidSafetyConfig.vi"("error in (no error)"=w65, "mode"=WPI_SafetyOutputConfigMenu."Enable", "SolenoidDevRef"=w66) -> ()  [unwired: 7 in, 2 out]
  n77 = call <vilib>:"WPI_SolenoidSafetyConfig.vi"("error in (no error)"=w11, "mode"=WPI_SafetyOutputConfigMenu."Enable", "SolenoidDevRef"=w10) -> ()  [unwired: 7 in, 2 out]
